vi "Referee.vi"(0 "element":u8[](array[numeric])) -> (4 "output cluster":T1, 15 "error out":errorcluster)   [LabVIEW 2017]
uses:
  SSL Referee.ctl
  SSL Referee Team Info.ctl
  Varint Decoder uint64.vi
  Varint Decoder uint32.vi
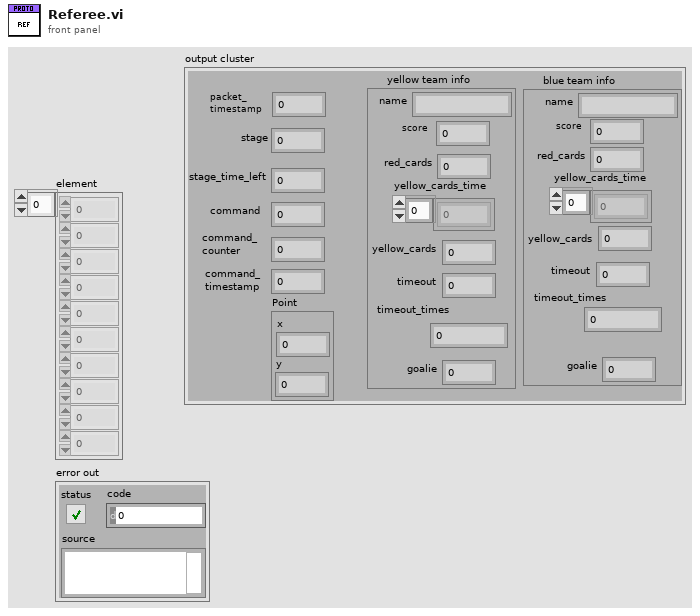
[diagram p1: front panel]
types:
  T1 = typedef "SSL Referee.ctl" = cluster{"packet_\ntimestamp":u64, "stage":u64, "stage_time_left":i32, "command ":u64, "command_\ncounter ":u32, "command_\ntimestamp":u64, "yellow team info":T2, "blue team info":T2, "Point":cluster{"x":sgl, "y":sgl}}
  T2 = typedef "SSL Referee Team Info.ctl" = cluster{"name":string, "score":u32, "red_cards":u32, "yellow_cards_time":u32[], "yellow_cards":u32, "timeout":u32, "timeout_times":u32, "goalie":u32}
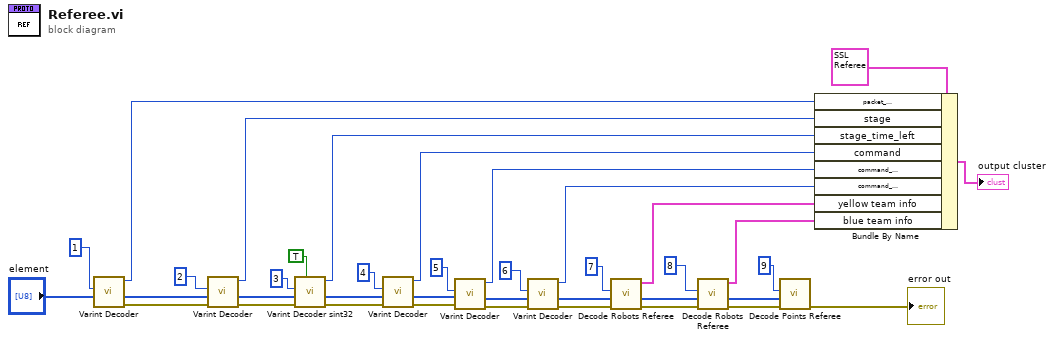
[diagram p0: block diagram]
diagram:
  n1 = call-poly "Varint Decoder.vi"("Array"="element", "Key"=1) -> ("error out"=w18:errorcluster, "array w/ subset deleted"=w16:u8[], "Varint"=w14:u64)  [unwired: 6 in, 1 out]
  n2 = call-poly "Varint Decoder.vi"("error in (no error)"=w18, "Array"=w16, "Key"=2) -> ("error out"=w21:errorcluster, "array w/ subset deleted"=w22:u8[], "Varint"=w13:u64)  [unwired: 5 in, 1 out]
  n3 = call "Varint Decoder sint32.vi"("Optional"=TRUE, "error in (no error)"=w21, "Array"=w22, "Key"=3) -> ("error out"=w24:errorcluster, "array w/ subset deleted"=w25:u8[], "Varint"=w12:i32)  [unwired: 4 in, 1 out]
  n4 = call-poly "Varint Decoder.vi"("error in (no error)"=w24, "Array"=w25, "Key"=4) -> ("error out"=w27:errorcluster, "array w/ subset deleted"=w29:u8[], "Varint"=w11:u64)  [unwired: 5 in, 1 out]
  n5 = call-poly "Varint Decoder.vi"("error in (no error)"=w27, "Array"=w29, "Key"=5) -> ("error out"=w28:errorcluster, "array w/ subset deleted"=w30:u8[], "Varint"=w10:u32)  [unwired: 5 in, 1 out]
  n6 = call-poly "Varint Decoder.vi"("error in (no error)"=w28, "Array"=w30, "Key"=6) -> ("error out"=w33:errorcluster, "array w/ subset deleted"=w35:u8[], "Varint"=w9:u64)  [unwired: 5 in, 1 out]
  n7 = call "Decode Robots Referee.vi"("error in"=w33, "array"=w35, "Key"=7) -> ("error out"=w34:errorcluster, "array w/ subset deleted out"=w36:u8[], "team info"=w8:T2)  [unwired: 6 in]
  n8 = call "Decode Robots Referee.vi"("error in"=w34, "array"=w36, "Key"=8) -> ("error out"=w6:errorcluster, "array w/ subset deleted out"=w4:u8[], "team info"=w7:T2)  [unwired: 6 in]
  n9 = call "Decode Points Referee.vi"("error in"=w6, "array"=w4, "Key"=9) -> ("error out"=→"error out":errorcluster)  [unwired: 6 in, 2 out]
  n10 = Bundle By Name(cluster=T1 {"packet_\ntimestamp"=0, "stage"=0, "stage_time_left"=0, "command "=0, "command_\ncounter "=0, "command_\ntimestamp"=0, "yellow team info"={"name"="", "score"=0, "red_cards"=0, "yellow_cards_time"=[], "yellow_cards"=0, "timeout"=0, "timeout_times"=0, "goalie"=0}, "blue team info"={"name"="", "score"=0, "red_cards"=0, "yellow_cards_time"=[], "yellow_cards"=0, "timeout"=0, "timeout_times"=0, "goalie"=0}, "Point"={"x"=0.0, "y"=0.0}} ("output cluster"), "packet_\ntimestamp"=w14, "stage"=w13, "stage_time_left"=w12, "command"=w11, "command_\ncounter"=w10, "command_\ntimestamp"=w9, "yellow team info"=w8, "blue team info"=w7) -> (→"output cluster":T1)
